vi "Create Waveforms.vi"() -> (2 "core pressure":dbl[](array[numeric]) format="%.2f", 4 "core temperature":dbl[](array[numeric]) format="%.2f")   [LabVIEW 2013]
doc: "This is a subVI used to create simulated data for the Database Tools examples named Logging Example, Logging Example (parameterized), and Parameterized. You specify the number of data points and two arrays of simulated core pressure and core temperature data are returned."
panel:
  in  "# of samples":i32=100
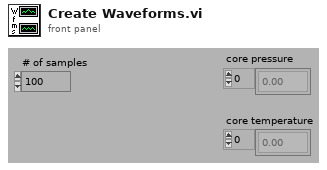
[diagram p1: front panel]
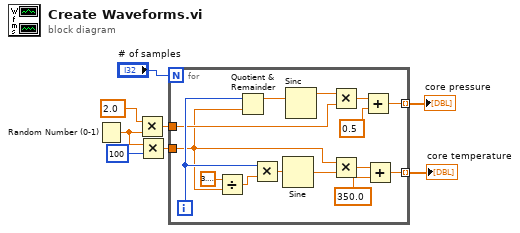
[diagram p0: block diagram]
diagram:
  n1 = Random Number (0-1)() -> (number: 0 to 1=w6:dbl)
  n2 = Multiply(x=2.0, y=w6) -> (x*y=w7:dbl)
  n3 = Multiply(x=w6, y=100) -> (x*y=w2:dbl)
  n4 = for {
    N: "# of samples" -> [_]
    tunnel: w7 -> [w15]
    tunnel: [w19] -> w4 mode=indexing
    tunnel: [w10] -> w5 mode=indexing
    tunnel: w2 -> [w12]
    i -> [w20]
    n5 = Divide(x=3.141592653589793, y=w12) -> (x/y=w14:dbl)
    n6 = Quotient & Remainder(x=w20, y=w12) -> (x-y*floor(x/y)=w22:dbl)  [unwired: 1 out]
    n7 = Multiply(x=w20, y=w14) -> (x*y=w21:dbl)
    n8 = Sine(x=w21) -> (sin(x)=w16:dbl)
    n9 = Sinc(1:w22) -> (0:w23:dbl)
    n10 = Multiply(x=w23, y=w15) -> (x*y=w11:dbl)
    n11 = Multiply(x=w12, y=w16) -> (x*y=w17:dbl)
    n12 = Add(x=w11, y=0.5) -> (x+y=w10:dbl)
    n13 = Add(x=w17, y=350.0) -> (x+y=w19:dbl)
  }
  "core temperature" <- w4
  "core pressure" <- w5
